vi "Time.vi"(8 "Wished Time":dbl, 9 "Reset":bool, 10 "Advance Time":bool, 11 "error in":errorcluster) -> (1 "Elapsed Time":dbl, 2 "Expired":bool, 3 "error out":errorcluster)   [LabVIEW 2024]
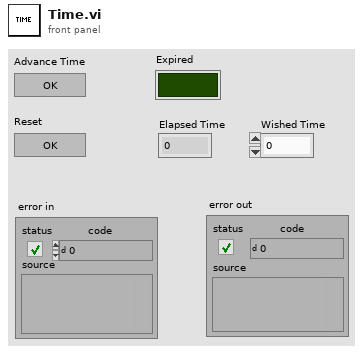
[diagram p1: front panel]
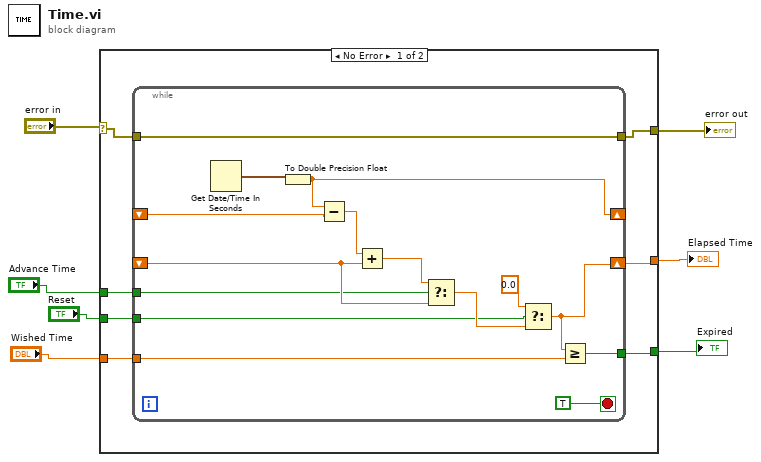
[diagram p0: block diagram]
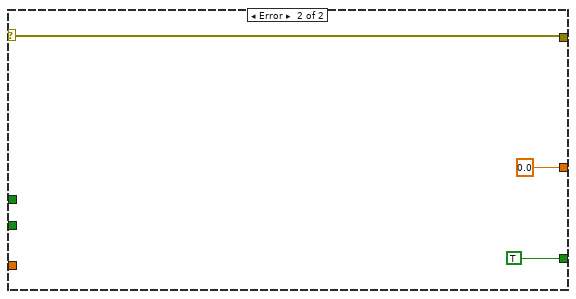
[diagram p2: hidden frame]
diagram:
  n1 = case shown="No Error" "error in" {
    selector: "error in" -> [w9 w30]
    tunnel: "Reset" -> [w14 _]
    tunnel: "Advance Time" -> [w13 _]
    tunnel: "Wished Time" -> [w12 _]
    tunnel: [w10 TRUE] -> w4
    tunnel: [w11 0.0 ("Elapsed Time")] -> w3
    tunnel: [w8 w30] -> w1
    frame No Error {
      n2 = while {
        shift-right: [w26] -> _
        shift-left: _ -> [w27]
        shift-right: [w22] -> w11
        shift-left: _ -> [w19]
        tunnel: [w21] -> w10
        tunnel: w14 -> [w20]
        tunnel: w13 -> [w18]
        tunnel: w12 -> [w17]
        tunnel: [w15] -> w8
        tunnel: w9 -> [w15]
        stop <- TRUE stop-if-true
        n3 = Get Date/Time In Seconds() -> (seconds since 1Jan1904=w29:timestamp)
        n4 = To Double Precision Float(number=w29) -> (double precision float=w26:dbl)
        n5 = Subtract(x=w26, y=w27) -> (x-y=w28:dbl)
        n6 = Add(x=w28, y=w19) -> (x+y=w25:dbl)
        n7 = Select(t=w25, s=w18, f=w19) -> (s? t:f=w24:dbl)
        n8 = Select(t=0.0, s=w20, f=w24) -> (s? t:f=w22:dbl)
        n9 = Greater Or Equal?(x=w22, y=w17) -> (x >= y?=w21:bool)
      }
    }
    frame Error {
    }
  }
  "Expired" <- w4
  "Elapsed Time" <- w3
  "error out" <- w1
